vi "dy_dt.vi"(8 "dt":dbl=1.0 format="%0.2f", 11 "y":dbl[](array[numeric])) -> (3 "dy/dt":dbl[](array[numeric]))   [LabVIEW 2013]
uses:
  <vilib>/Analysis/NI_AALPro.lvlib
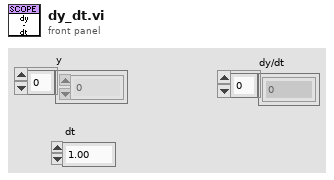
[diagram p1: front panel]
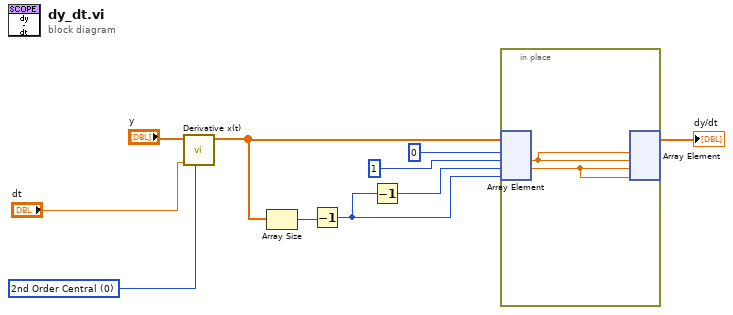
[diagram p0: block diagram]
diagram:
  w10 = u16 0 items=["2nd Order Central", "4th Order Central", "Forward", "Backward"] ("method")
  n1 = call <vilib>:"Derivative x(t).vi"("method"=w10, "dt"="dt", "X"="y") -> ("dX/dt"=w9:dbl[])  [unwired: 7 in, 1 out]
  n2 = Array Size(array=w9) -> (size(s)=w8:i32)
  n3 = Decrement(x=w8) -> (x-1=w2:i32)
  n4 = Decrement(x=w2) -> (x-1=w7:i32)
  n5 = in-place {
    n6 = in-place-array #1(w9, 0, 1, w7, w2) -> (w12:dbl, w11:dbl)  [unwired: 2 out]
    n7 = in-place-array #1(w12, w12, w11, w11) -> (→"dy/dt":dbl[])  [unwired: 4 out]
  }
